vi "Set Manual Volt per Division.vi"(8 "error in (no error)":errorcluster, 9 "V/div":T1, 11 "MSOX6004 in":refnum<class "MSOX6004.lvclass">) -> (0 "error out":errorcluster, 3 "MSOX6004 out":refnum<class "MSOX6004.lvclass">)   [LabVIEW 2018, in "MSOX6004.lvlib" / "MSOX6004.lvclass"]
uses:
  MSOX6004.lvclass
  PPLs/Oscilloscope/Parent/Oscilloscope.lvlibp/Custom Controls/Volts per Division.ctl
  PPLs/Oscilloscope/Parent/Oscilloscope.lvlibp/Custom Controls/Analog Channels.ctl
  MSOX6004.lvclass/MSOX6004.ctl
  <instrlib>/Keysight InfiniiVision/Keysight InfiniiVision.lvlib
  PPLs/Oscilloscope/Parent/Oscilloscope.lvlibp
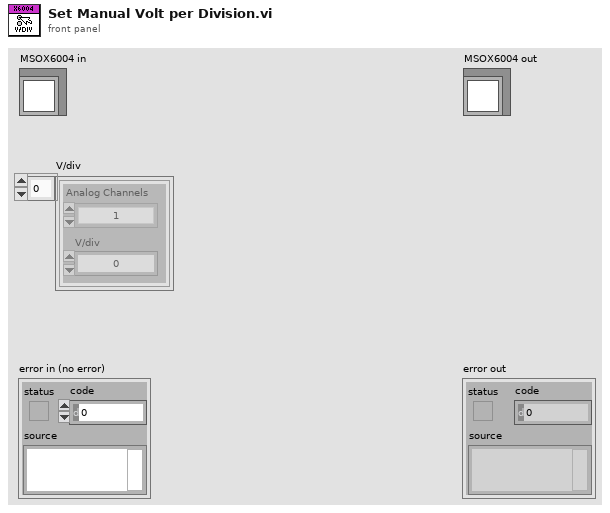
[diagram p1: front panel]
types:
  T1 = typedef "Oscilloscope.lvlibp/Volts per Division.ctl" = cluster{"Analog Channels":T2, "V/div":dbl}[]
  T2 = typedef "Oscilloscope.lvlibp/Analog Channels.ctl" = enum16{"1", "2", "3", "4", "5", "6", "7", "8", "9", "10", "11", "12", "13", "14", "15", "16"}
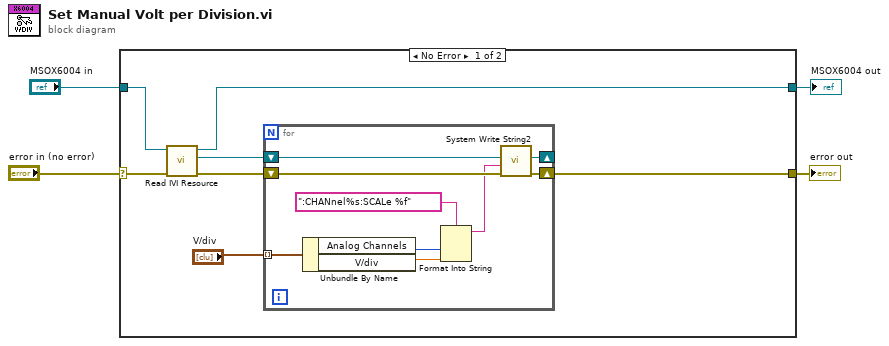
[diagram p0: block diagram]
diagram:
  n1 = case shown="No Error" "error in (no error)" {
    selector: "error in (no error)" -> [w11 w22]
    tunnel: [w5 w22] -> w1
    tunnel: [w8 w21] -> w2
    tunnel: "MSOX6004 in" -> [w10 w21]
    frame No Error {
      n2 = call "Read IVI Resource.vi"("error in (no error)"=w11, "MSOX6004 in"=w10) -> ("error out"=w9:errorcluster, "IVI Resource"=w7:refnum<k15>, "MSOX6004 out"=w8:refnum<class "MSOX6004.lvclass">)  [unwired: 7 in]
      n3 = for {
        tunnel: "V/div" -> [w20] mode=indexing
        shift-right: [w18] -> w5
        shift-left: w9 -> [w19]
        shift-right: [w12] -> _
        shift-left: w7 -> [w17]
        n4 = Unbundle By Name(w20) -> ("Analog Channels"=w15:T2, "V/div"=w14:dbl)
        n5 = Format Into String(format string=":CHANnel%s:SCALe %f", w15, w14) -> (resulting string=w13:string)  [unwired: 2 in, 1 out]
        n6 = call <instrlib>:"System Write String2.vi"("error in (no error)"=w19, "Data"=w13, "instrument handle"=w17) -> ("error out"=w18:errorcluster, "instrument handle out"=w12:refnum<k15>)  [unwired: 7 in]
      }
    }
    frame Error {
    }
  }
  "error out" <- w1
  "MSOX6004 out" <- w2
